vi "ParseSlaveRY.vi"(0 "RY":bool[][](array[boolean])) -> (2 "PLC状态":T1)   [LabVIEW 2018]
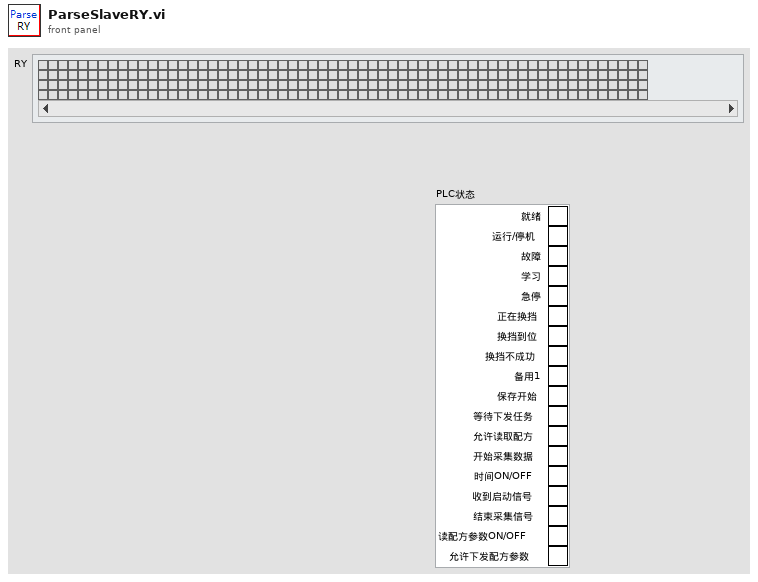
[diagram p1: front panel]
types:
  T1 = cluster{"就绪":bool, "运行/停机":bool, "故障":bool, "学习":bool, "急停":bool, "正在换挡":bool, "换挡到位":bool, "换挡不成功":bool, "备用1":bool, "保存开始":bool, "等待下发任务":bool, "允许读取配方":bool, "开始采集数据":bool, "时间ON/OFF":bool, " 收到启动信号":bool, "结束采集信号":bool, "读配方参数ON/OFF":bool, "允许下发配方参数":bool}
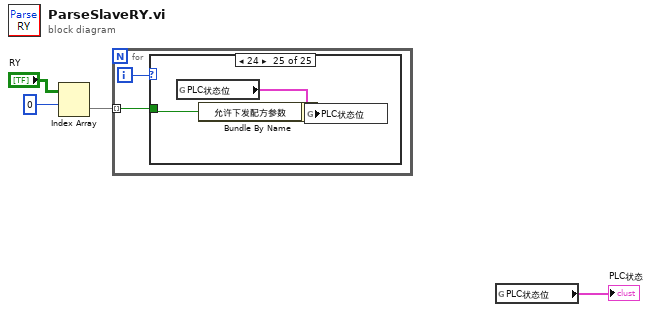
[diagram p0: block diagram]
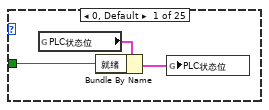
[diagram p2: hidden frame]
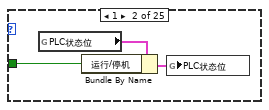
[diagram p3: hidden frame]
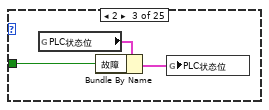
[diagram p4: hidden frame]
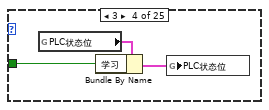
[diagram p5: hidden frame]
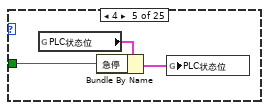
[diagram p6: hidden frame]
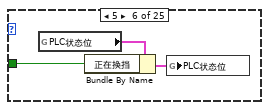
[diagram p7: hidden frame]
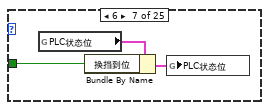
[diagram p8: hidden frame]
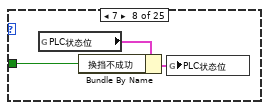
[diagram p9: hidden frame]
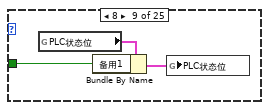
[diagram p10: hidden frame]
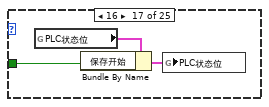
[diagram p18: hidden frame]
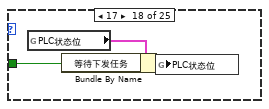
[diagram p19: hidden frame]
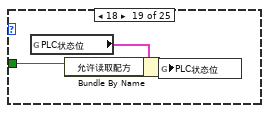
[diagram p20: hidden frame]
diagram:
  n1 = Index Array(array="RY", index (row)=0 ("索引 (行)")) -> (element=w2:bool[])  [unwired: 1 in]
  n2 = for {
    tunnel: w2 -> [w5] mode=indexing
    i -> [w6]
    n3 = case shown="24" w6 {
      tunnel: w5 -> [w8 w11 w14 w17 w20 w23 w26 w29 w32 _ _ _ _ _ _ _ w34 w37 w40 w43 w46 w49 w52 w55 w58]
      frame 0, Default {
        n4 = global read "全局 1.vi" "PLC状态位"() -> (w9:T1)
        n5 = Bundle By Name(cluster=w9, "就绪"=w8) -> (w7:T1)
        n6 = global write "全局 1.vi" "PLC状态位"(w7) -> ()
      }
      frame 1 {
        n7 = global read "全局 1.vi" "PLC状态位"() -> (w12:T1)
        n8 = Bundle By Name(cluster=w12, "运行/停机"=w11) -> (w10:T1)
        n9 = global write "全局 1.vi" "PLC状态位"(w10) -> ()
      }
      frame 2 {
        n10 = global read "全局 1.vi" "PLC状态位"() -> (w15:T1)
        n11 = Bundle By Name(cluster=w15, "故障"=w14) -> (w13:T1)
        n12 = global write "全局 1.vi" "PLC状态位"(w13) -> ()
      }
      frame 3 {
        n13 = global read "全局 1.vi" "PLC状态位"() -> (w18:T1)
        n14 = Bundle By Name(cluster=w18, "学习"=w17) -> (w16:T1)
        n15 = global write "全局 1.vi" "PLC状态位"(w16) -> ()
      }
      frame 4 {
        n16 = global read "全局 1.vi" "PLC状态位"() -> (w21:T1)
        n17 = Bundle By Name(cluster=w21, "急停"=w20) -> (w19:T1)
        n18 = global write "全局 1.vi" "PLC状态位"(w19) -> ()
      }
      frame 5 {
        n19 = global read "全局 1.vi" "PLC状态位"() -> (w24:T1)
        n20 = Bundle By Name(cluster=w24, "正在换挡"=w23) -> (w22:T1)
        n21 = global write "全局 1.vi" "PLC状态位"(w22) -> ()
      }
      frame 6 {
        n22 = global read "全局 1.vi" "PLC状态位"() -> (w27:T1)
        n23 = Bundle By Name(cluster=w27, "换挡到位"=w26) -> (w25:T1)
        n24 = global write "全局 1.vi" "PLC状态位"(w25) -> ()
      }
      frame 7 {
        n25 = global read "全局 1.vi" "PLC状态位"() -> (w30:T1)
        n26 = Bundle By Name(cluster=w30, "换挡不成功"=w29) -> (w28:T1)
        n27 = global write "全局 1.vi" "PLC状态位"(w28) -> ()
      }
      frame 8 {
        n28 = global read "全局 1.vi" "PLC状态位"() -> (w33:T1)
        n29 = Bundle By Name(cluster=w33, "备用1"=w32) -> (w31:T1)
        n30 = global write "全局 1.vi" "PLC状态位"(w31) -> ()
      }
      frame 9 {
      }
      frame 10 {
      }
      frame 11 {
      }
      frame 12 {
      }
      frame 13 {
      }
      frame 14 {
      }
      frame 15 {
      }
      frame 16 {
        n31 = global read "全局 1.vi" "PLC状态位"() -> (w36:T1)
        n32 = Bundle By Name(cluster=w36, "保存开始"=w34) -> (w35:T1)
        n33 = global write "全局 1.vi" "PLC状态位"(w35) -> ()
      }
      frame 17 {
        n34 = global read "全局 1.vi" "PLC状态位"() -> (w39:T1)
        n35 = Bundle By Name(cluster=w39, "等待下发任务"=w37) -> (w38:T1)
        n36 = global write "全局 1.vi" "PLC状态位"(w38) -> ()
      }
      frame 18 {
        n37 = global read "全局 1.vi" "PLC状态位"() -> (w42:T1)
        n38 = Bundle By Name(cluster=w42, "允许读取配方"=w40) -> (w41:T1)
        n39 = global write "全局 1.vi" "PLC状态位"(w41) -> ()
      }
      frame 19 {
        n40 = global read "全局 1.vi" "PLC状态位"() -> (w45:T1)
        n41 = Bundle By Name(cluster=w45, "开始采集数据"=w43) -> (w44:T1)
        n42 = global write "全局 1.vi" "PLC状态位"(w44) -> ()
      }
      frame 20 {
        n43 = global read "全局 1.vi" "PLC状态位"() -> (w48:T1)
        n44 = Bundle By Name(cluster=w48, "时间ON/OFF"=w46) -> (w47:T1)
        n45 = global write "全局 1.vi" "PLC状态位"(w47) -> ()
      }
      frame 21 {
        n46 = global read "全局 1.vi" "PLC状态位"() -> (w51:T1)
        n47 = Bundle By Name(cluster=w51, "收到启动信号"=w49) -> (w50:T1)
        n48 = global write "全局 1.vi" "PLC状态位"(w50) -> ()
      }
      frame 22 {
        n49 = global read "全局 1.vi" "PLC状态位"() -> (w54:T1)
        n50 = Bundle By Name(cluster=w54, "结束采集信号"=w52) -> (w53:T1)
        n51 = global write "全局 1.vi" "PLC状态位"(w53) -> ()
      }
      frame 23 {
        n52 = global read "全局 1.vi" "PLC状态位"() -> (w57:T1)
        n53 = Bundle By Name(cluster=w57, "读配方参数ON/OFF"=w55) -> (w56:T1)
        n54 = global write "全局 1.vi" "PLC状态位"(w56) -> ()
      }
      frame 24 {
        n55 = global read "全局 1.vi" "PLC状态位"() -> (w60:T1)
        n56 = Bundle By Name(cluster=w60, "允许下发配方参数"=w58) -> (w59:T1)
        n57 = global write "全局 1.vi" "PLC状态位"(w59) -> ()
      }
    }
  }
  n58 = global read "全局 1.vi" "PLC状态位"() -> (→"PLC状态":T1)
